vi "Update Generic Counter Value.vi"(8 "Increment?":bool, 11 "Input Counter Val":u16) -> (3 "Updated Counter Val":u16)   [LabVIEW 2014]
panel:
  # "Copyright 2014 Vidrio Technologies\nScanImage 5 software is licensed under the Apache License, Version 2.0 (the \"License\"); you may not use any files contained\nwithin the ScanImage 5 release except in compliance with the License. You may obtain a copy of the License at\n http://www.apache.org/licenses/LICENSE-2.0\nUnless required by applicable law or agreed to in writing, software distributed under the License is distributed on an\n\"AS IS\" BASIS, WITHOUT WARRANTIES OR CONDITIONS OF ANY KIND, either express or implied. See the License for the\n specific language governing permissions and limitations under the License."
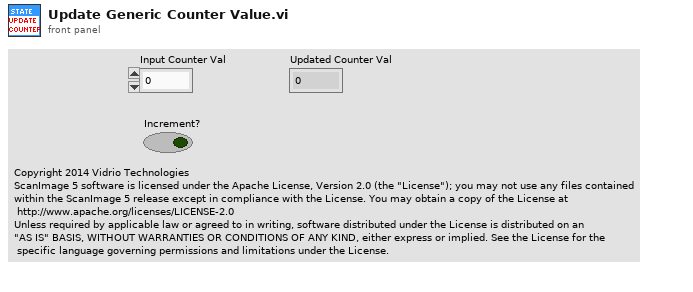
[diagram p1: front panel]
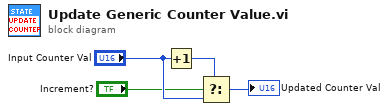
[diagram p0: block diagram]
diagram:
  n1 = Increment(x="Input Counter Val") -> (x+1=w4:u16)
  n2 = Select(t=w4, s="Increment?", f="Input Counter Val") -> (s? t:f=→"Updated Counter Val":u16)
